vi "rotm_to_euler.vi"(1 "Rotation Matrix":T1) -> (0 "Orientation XYZ":dbl[](array[numeric]))   [LabVIEW 2019]
uses:
  <vilib>/Analysis/Matrix/Datatypes/RealMatrix.ctl
  <vilib>/Analysis/Matrix/NI_Matrix.lvlib
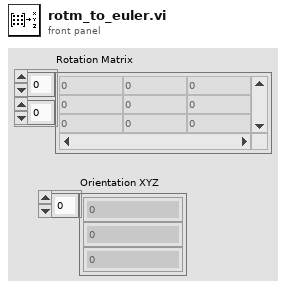
[diagram p1: front panel]
types:
  T1 = typedef "NI_Matrix.lvlib/RealMatrix.ctl" = dbl[][]
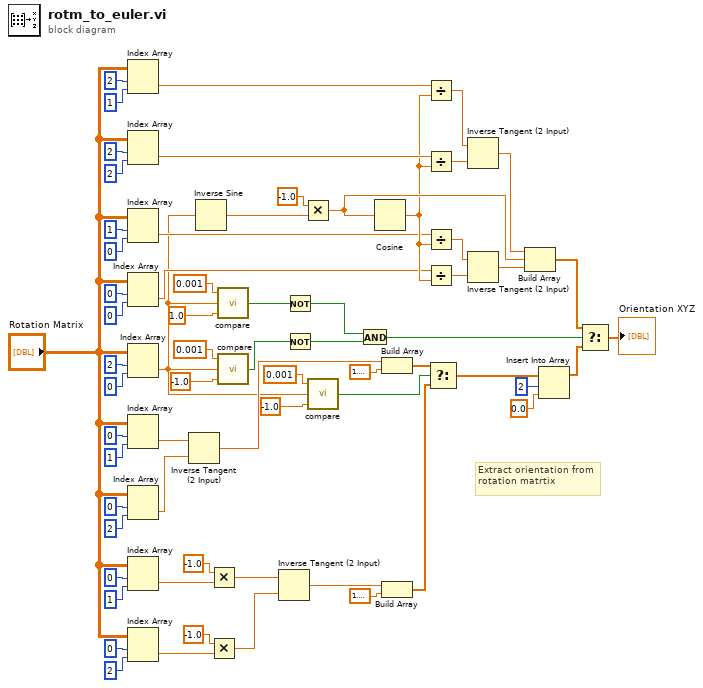
[diagram p0: block diagram]
diagram:
  # "Extract orientation from rotation matrtix"
  n1 = Index Array(array="Rotation Matrix", index (row)=2, index (col)=1) -> (element=w58:dbl)
  n2 = Index Array(array="Rotation Matrix", index (row)=2, index (col)=2) -> (element=w57:dbl)
  n3 = Index Array(array="Rotation Matrix", index (row)=1, index (col)=0) -> (element=w47:dbl)
  n4 = Index Array(array="Rotation Matrix", index (row)=0, index (col)=0) -> (element=w44:dbl)
  n5 = Index Array(array="Rotation Matrix", index (row)=2, index (col)=0) -> (element=w3:dbl)
  n6 = Index Array(array="Rotation Matrix", index (row)=0, index (col)=1) -> (element=w34:dbl)
  n7 = Index Array(array="Rotation Matrix", index (row)=0, index (col)=2) -> (element=w33:dbl)
  n8 = Index Array(array="Rotation Matrix", index (row)=0, index (col)=1) -> (element=w25:dbl)
  n9 = Index Array(array="Rotation Matrix", index (row)=0, index (col)=2) -> (element=w19:dbl)
  n10 = Inverse Tangent (2 Input)(1:w33, 2:w34) -> (0:w35:dbl)
  n11 = Inverse Sine(1:w3) -> (0:w63:dbl)
  n12 = Multiply(x=-1.0, y=w25) -> (x*y=w22:dbl)
  n13 = Multiply ("Multiply.vi")(x=-1.0, y=w19) -> (x*y=w21:dbl)
  n14 = call "compare.vi"("Value 2"=1.0, "Value 1"=w3, "Tolerance"=0.001) -> ("Comparison"=w9:bool)
  n15 = call "compare.vi"("Value 2"=-1.0, "Value 1"=w3, "Tolerance"=0.001) -> ("Comparison"=w7:bool)
  n16 = Inverse Tangent (2 Input)(1:w21, 2:w22) -> (0:w24:dbl)
  n17 = Not(x=w9) -> (.not. x?=w8:bool)
  n18 = Not(x=w7) -> (.not. x?=w6:bool)
  n19 = Multiply(x=-1.0, y=w63) -> (x*y=w52:dbl)
  n20 = call "compare.vi"("Value 2"=-1.0, "Value 1"=w3, "Tolerance"=0.001) -> ("Comparison"=w5:bool)
  n21 = And(x=w8, y=w6) -> (x .and. y?=w10:bool)
  n22 = Cosine(x=w52) -> (cos(x)=w48:dbl)
  n23 = Build Array(w35, 1.5707963267948966) -> (w37:dbl[])
  n24 = Build Array(w24, 1.5707963267948966) -> (w36:dbl[])
  n25 = Divide(x=w58, y=w48) -> (x/y=w59:dbl)
  n26 = Divide(x=w57, y=w48) -> (x/y=w56:dbl)
  n27 = Divide(x=w47, y=w48) -> (x/y=w50:dbl)
  n28 = Divide(x=w44, y=w48) -> (x/y=w49:dbl)
  n29 = Select(t=w37, s=w5, f=w36) -> (s? t:f=w41:dbl[])
  n30 = Inverse Tangent (2 Input)(1:w56, 2:w59) -> (0:w53:dbl)
  n31 = Inverse Tangent (2 Input)(1:w49, 2:w50) -> (0:w51:dbl)
  n32 = Build Array(w53, w52, w51) -> (w64:dbl[])
  n33 = Insert Into Array(array=w41, index=2, new element=0.0 ("element")) -> (w38:dbl[])
  n34 = Select(t=w64, s=w10, f=w38) -> (s? t:f=→"Orientation XYZ":dbl[])
